vi "6 Comp Balance Global.vi"() -> ()   [LabVIEW 2021]
panel:
  in  "Current Values":dbl[](array[numeric])
  out "End ms":u32
  out "Start ms":u32
  in  "Balance Data":dbl[][](array[numeric])
  in  "Channels to Log":i32[](array[numeric])
  in  "Take Balance data":bool
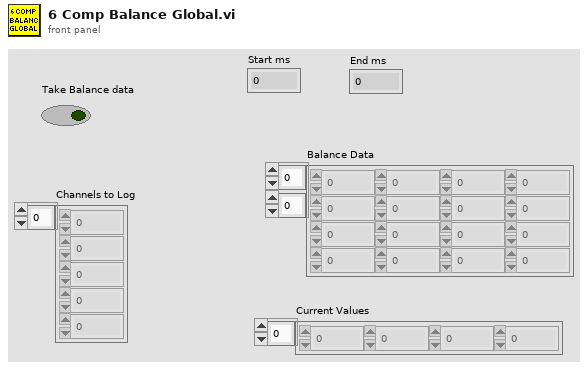
[diagram p1: front panel]
diagram:
